vi "运维调试_氨氮.vi"() -> ()   [LabVIEW 2016, in "氨氮.lvlib"]
uses:
  <vilib>/Platform/TimedLoop/XDataNode/timing_clust.ctl
  <vilib>/Platform/TimedLoop/XDataNode/nitl_modes.ctl
  <vilib>/Platform/TimedLoop/XDataNode/wakeup.ctl
  <vilib>/Utility/miscctls.llb/LVPointTypeDef.ctl
  <vilib>/Platform/TimedLoop/XDataNode/XDataNode.xnode
  <vilib>/Platform/TimedLoop/XDataNode/XDNodeRunTimeDep.lvlib
panel:
  out "固件版本号":string
  in  "数组":string[](array[string])
  in  "备用系数写入":bool
  in  "备用系数读取":bool
  in  "备用系数":T1
  in  "量程切换阈值写入":bool
  in  "量程切换阈值读取":bool
  in  "量程切换阈值":cluster{"阈值":dbl, "标液浓度":dbl}
  in  "参数下拉列表":enum16{"氨氮", "总磷"}(ring)
  in  "量程下拉列表":enum16{"低量程", "高量程"}(ring)
  in  "测量模式下拉列表":enum16{"水样测量", "空白核查", "标样核查", "盲样测试", "加标回收"}(ring)
  in  "公式":cluster{"X^2":dbl, "X":dbl, "b":dbl}
  in  "写公式":bool
  in  "读公式":bool
  in  "精度":dbl=4.0
  in  "样品5 F0":dbl
  in  "样品5 F1":dbl
  in  "样品4 F1":dbl
  in  "样品4 F0":dbl
  in  "样品3 F0":dbl
  in  "样品3 F1":dbl
  in  "样品2 F0":dbl
  in  "样品2 F1":dbl
  in  "样品1 F1":dbl
  in  "样品1 F0":dbl
  in  "method":u16(ring) items=["最小二乘", "最小绝对残差", "Bisquare"]
  in  "模型":enum32{"线性", "多项式"}(ring)
  out "r^2":dbl format="%.7g"
  out "拟合公式":string
  in  "样品2启用":bool
  in  "样品5启用":bool
  in  "样品4启用":bool
  in  "样品3启用":bool
  in  "样品1启用":bool
  in  "标液浓度5":dbl
  in  "测量吸光度5":dbl
  in  "标液浓度4":dbl
  in  "测量吸光度4":dbl
  in  "标液浓度3":dbl
  in  "测量吸光度3":dbl
  in  "标液浓度2":dbl
  in  "测量吸光度2":dbl
  in  "测量吸光度1":dbl
  in  "标液浓度1":dbl
  out "XY图":cluster{"X Values":dbl[], "Y Values":dbl[]}[](graph)
  in  "返回":bool
  in  "设置":bool
  out "序列号":string="序列号"
  out "氨氮测量数据":T2(xcontrol)
  out "集成报警信息":string
  out "设置值":dbl
  out "定时启动":bool
  out "总磷总氮运行状态":T3(xcontrol)
  in  "停止":bool
  in  "手动启动":bool
  in  "单步测试":bool
  in  "总磷氨氮调试":u16[](xcontrol)
  out "F3":sgl format="%#.6f"
  out "F2":sgl format="%#.6f"
  out "F1":sgl format="%#.6f"
  out "F0":sgl format="%#.6f"
  out "多列列表框":i32(listbox)
  # "COM6"
  # "参数设置"
  # "标液浓度"
  # "F0"
  # "F1"
  # "吸光值显示"
  # "样品一"
  # "辅\n助\n计\n算\n区"
  # "样品二"
  # "样品三"
  # "样品四"
  # "样品五"
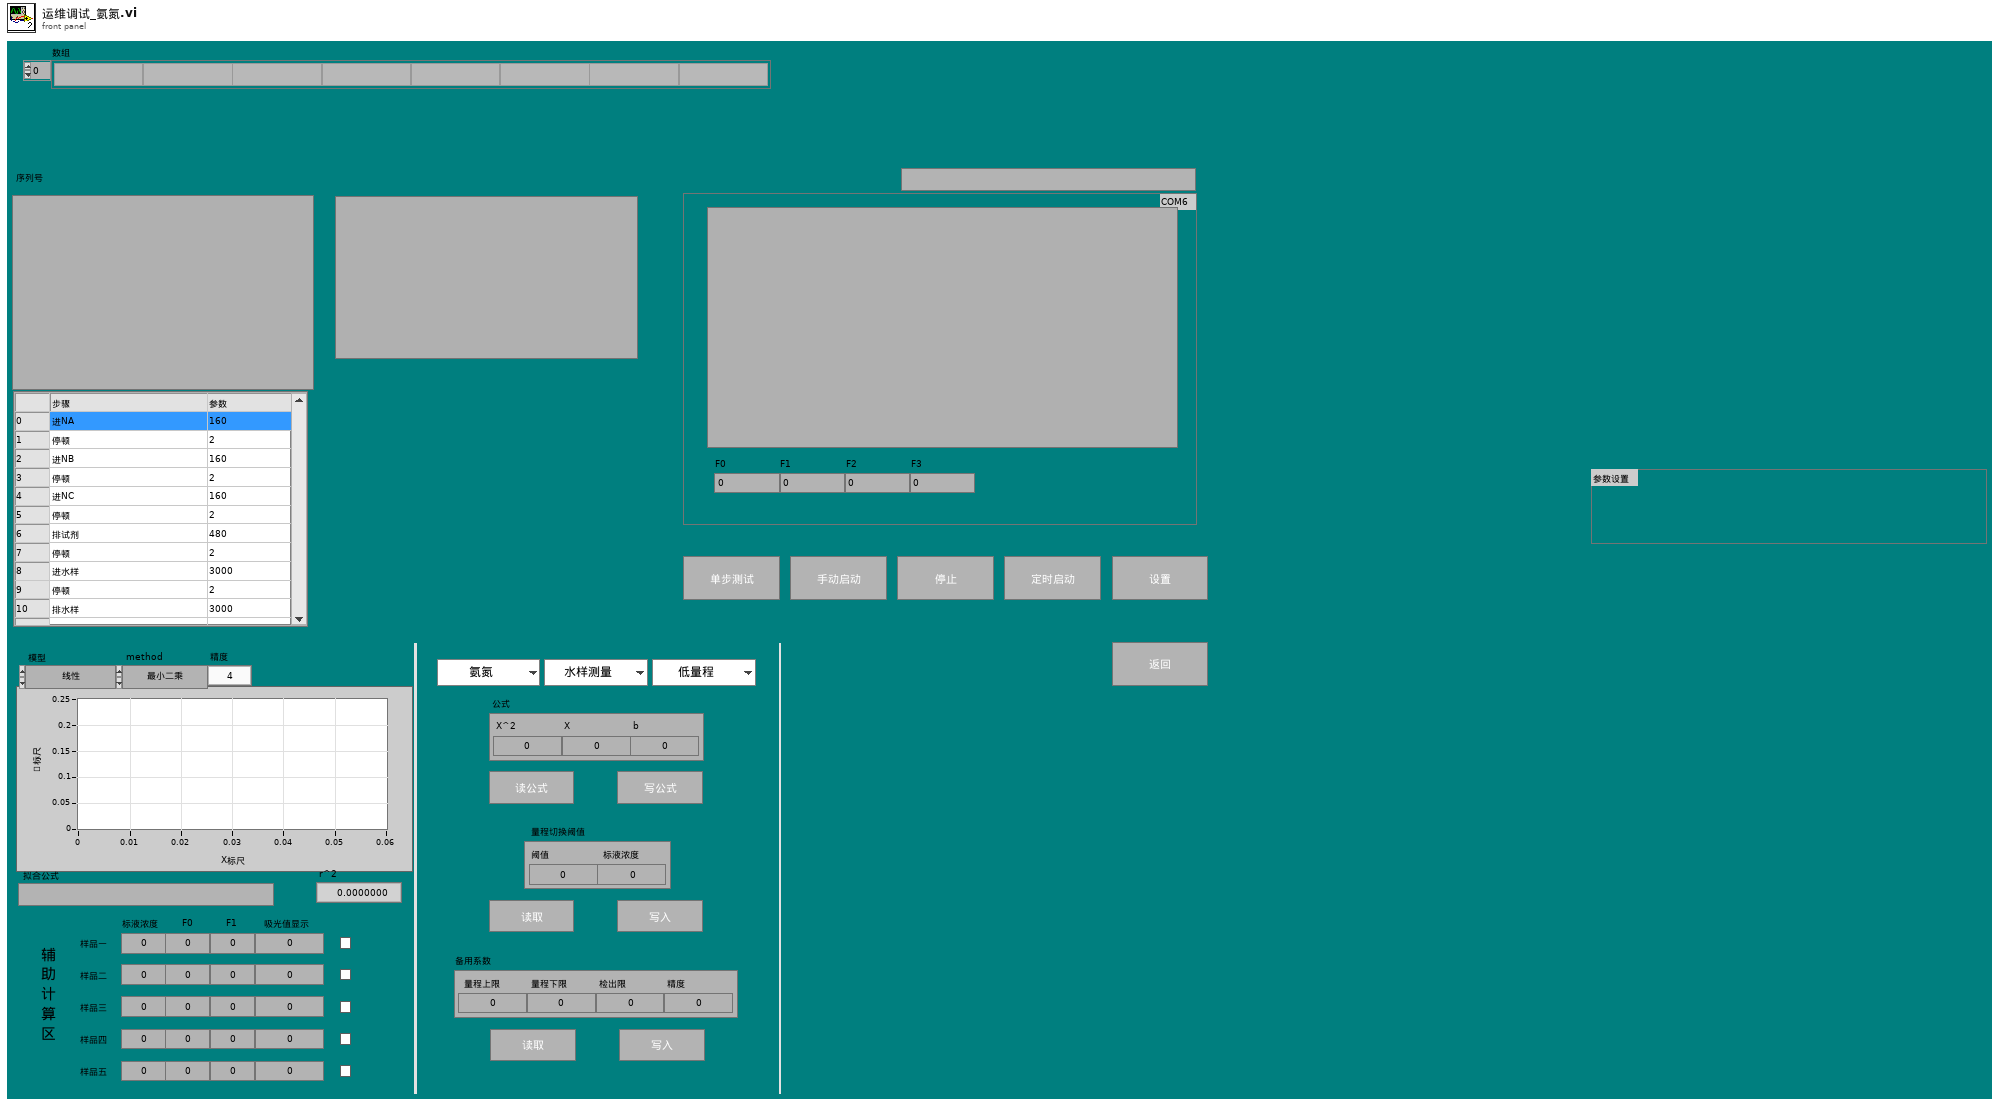
[diagram p1: front panel]
types:
  T1 = cluster{"量程上限":dbl, "量程下限":dbl, "检出限":dbl, "精度":dbl}
  T2 = cluster{"flowid":u16, "测量精度":u16, "测量数据区":cluster{"因子编码":u32, "单位":u16, "标样参考值":sgl, "水样数据时间":timestamp, "水样实测值":sgl, "水样数据标识":string, "标样数据时间":timestamp, "标样实测值":sgl, "标样数据标识":string, "空白数据时间":timestamp, "空白实测值":sgl, "空白数据标识":string, "零点核查数据时间":timestamp, "零点核查实测值":sgl, "零点核查数据标识":string, "跨度核查数据时间":timestamp, "跨度核查实测值":sgl, "跨度核查数据标识":string, "加标回收数据时间":timestamp, "加标回收实测值":sgl, "加标回收数据标识":string, "平行样数据时间":timestamp, "平行样实测值":sgl, "平行样数据标识":string}}
  T3 = cluster{"系统时间":timestamp, "工作状态":enum16{"空闲", "水样测试", "标样核查", "零点核查", "跨度核查", "空白测试", "平行样测试", "加标回收", "空白校准", "标样校准", "初始化（清洗）"}, "测量模式":enum16{"待机", "连续模式", "周期模式", "定点模式", "受控模式", "手动模式"}, "告警代码":enum16{"无告警", "缺试剂告警", "缺水样告警", "缺蒸馏水告警", "缺标液告警", "仪表漏液告警", "标定异常告警", "超量程告警", "加热异常", "低试剂预警", "超上限告警", "超下限告警", "仪表内部其他异常", "滴定异常告警", "电极异常告警", "量程切换告警", "参数设置告警", "PH电极电位异常", "电导率电极异常", "浊度光度异常", "溶解氧电极异常", "溶解氧光强异常", "温度异常告警", "PH异常告警", "溶解氧异常告警", "电导率异常告警", "浊度异常告警", "叶绿素异常告警", "藻密度异常告警", "蓝绿藻异常告警", "ORP异常告警", "氨氮异常告警", "清洁刷异常告警", "SD卡异常告警", "蓝牙异常告警", "Wifi异常告警", "流程异常告警"}, "故障代码":enum16{"无故障", "电机故障", "温度故障", "通讯故障", "滴定故障"}, "日志代码":u16, "软件版本":u16, "F0":sgl, "F1":sgl, "F2":sgl, "F3":sgl, "T":sgl, "H":sgl, "id":u16, "flowid":u16, "量程":u16}
  T4 = enum16{"待机", "启动氨氮", "氨氮测量中", "启动总磷", "总磷测量中", "延时"}
  T5 = typedef "LVPointTypeDef.ctl" = cluster{"Horizontal":i16, "Vertical":i16}
  T6 = cluster{"因子编码":u32, "单位":u16, "标样参考值":sgl, "水样数据时间":timestamp, "水样实测值":sgl, "水样数据标识":string, "标样数据时间":timestamp, "标样实测值":sgl, "标样数据标识":string, "空白数据时间":timestamp, "空白实测值":sgl, "空白数据标识":string, "零点核查数据时间":timestamp, "零点核查实测值":sgl, "零点核查数据标识":string, "跨度核查数据时间":timestamp, "跨度核查实测值":sgl, "跨度核查数据标识":string, "加标回收数据时间":timestamp, "加标回收实测值":sgl, "加标回收数据标识":string, "平行样数据时间":timestamp, "平行样实测值":sgl, "平行样数据标识":string}
  T7 = enum16{"空闲", "水样测试", "标样核查", "零点核查", "跨度核查", "空白测试", "平行样测试", "加标回收", "空白校准", "标样校准", "初始化（清洗）"}
  T8 = cluster{"启动模式":enum16{"标液测量", "水样测量", "零液测量", "盲样测量", "加标回收"}, "启动参数":u16, "量程":enum16{"低量程", "高量程"}}
  T9 = cluster{"时间标识":timestamp, "设备":string, "日志信息":string, "流程参数":string}
  T10 = cluster{"时间标识":timestamp, "设备":string, "日志信息":string}
  T11 = enum16{"无告警", "缺试剂告警", "缺水样告警", "缺蒸馏水告警", "缺标液告警", "仪表漏液告警", "标定异常告警", "超量程告警", "加热异常", "低试剂预警", "超上限告警", "超下限告警", "仪表内部其他异常", "滴定异常告警", "电极异常告警", "量程切换告警", "参数设置告警", "PH电极电位异常", "电导率电极异常", "浊度光度异常", "溶解氧电极异常", "溶解氧光强异常", "温度异常告警", "PH异常告警", "溶解氧异常告警", "电导率异常告警", "浊度异常告警", "叶绿素异常告警", "藻密度异常告警", "蓝绿藻异常告警", "ORP异常告警", "氨氮异常告警", "清洁刷异常告警", "SD卡异常告警", "蓝牙异常告警", "Wifi异常告警", "流程异常告警"}
  T12 = typedef "LVRowAndColumnUnsignedTypeDef.ctl" = cluster{"Row":u32, "Column":u32}
  T13 = typedef "XDNodeRunTimeDep.lvlib/timing_clust.ctl" = cluster{"Expected End [f-1]":u64, "Actual End [f-1]":u64, "Finished Late? [f-1]":bool, "Expected End [i-1]":u64, "Actual End [i-1]":u64, "Finished Late? [i-1]":bool, "Expected Start [i]":u64, "Actual Start [i]":u64, "Expected Start [f]":u64, "Actual Start [f]":u64, "Source Name":string, "Structure Name":string, "Period":i64, "Deadline":i64, "Offset":i64, "Start":i64, "Priority":i32, "Timeout":i32, "Mode":T14, "Wakeup Reason":T15, "Error":errorcluster, "Source Type":string, "Secondary Source Type":string, "Global End Time":u64, "Global Start Time":u64, "Frame Duration":u64, "Iteration Duration":u64, "Assigned CPU":i32, "I/O Scan Engine Mode":u32}
  T14 = typedef "XDNodeRunTimeDep.lvlib/nitl_modes.ctl" = enum32{"No Change", "Process missed periods, maintain original phase", "Discard missed periods, maintain original phase", "Process missed periods, ignore original phase", "Discard missed periods, ignore original phase"}
  T15 = typedef "XDNodeRunTimeDep.lvlib/wakeup.ctl" = enum32{"Normal", "Aborted", "Asynchronous wakeup", "Timing source error", "Timed loop error", "Timeout"}
  T16 = cluster{"站号":u16, "量程切换":enum32{"H", "L", "AUTO"}, "控制命令":enum16{"启动测量", "标样核查", "零点核查", "跨度核查", "空白测试", "平行样测试", "加标回收", "空白校准", "标样校准", "初始化（清洗）", "停止测试", "仪器重启", "校时", "模式设置", "测量间隔设置", "盲样测试"}, "模式设置":enum16{"待机", "连续模式", "周期模式", "定点模式", "受控模式", "手动模式"}, "测量间隔":u16}
  T17 = cluster{"站号":u16, "量程切换":enum32{"H", "L", "AUTO"}, "控制命令":enum16{"启动测量", "标样核查", "零点核查", "跨度核查", "空白测试", "平行样测试", "加标回收", "空白校准", "标样校准", "初始化（清洗）", "停止测试", "仪器重启", "校时", "模式设置", "测量间隔设置"}, "模式设置":enum16{"待机", "连续模式", "周期模式", "定点模式", "受控模式", "手动模式"}, "测量间隔":u16}
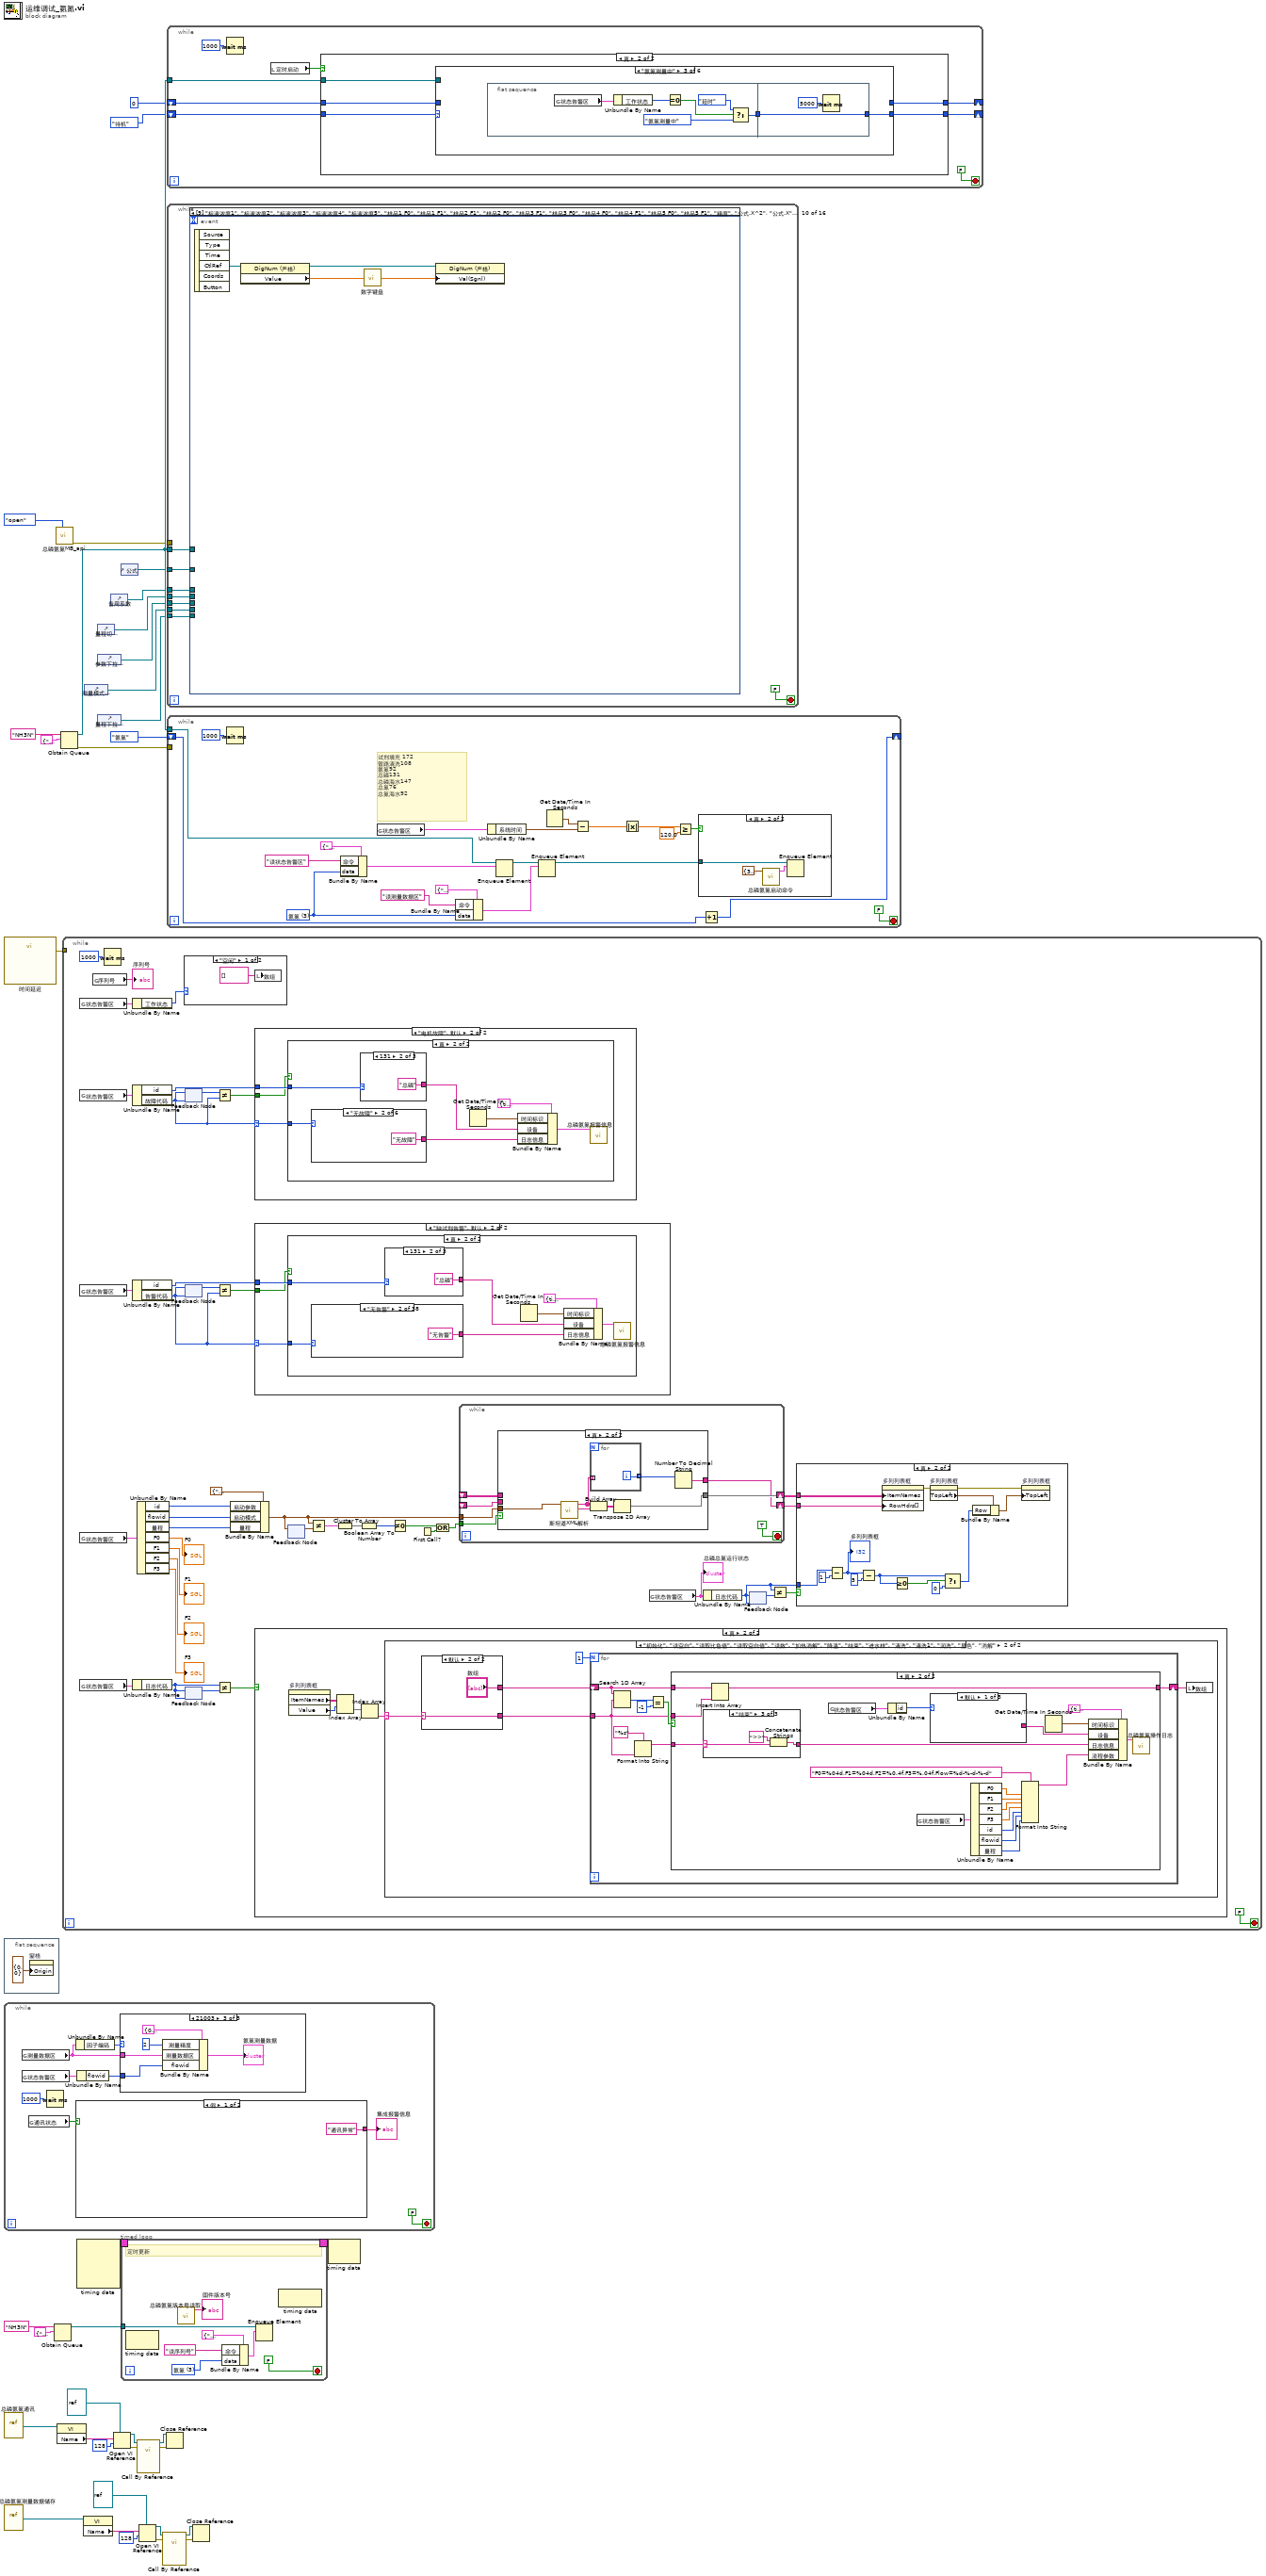
[diagram p0: block diagram]
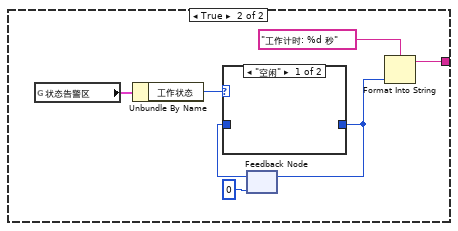
[diagram p2: hidden frame]
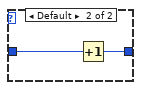
[diagram p3: hidden frame]
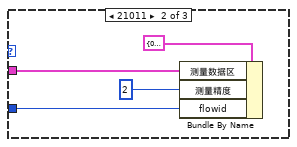
[diagram p5: hidden frame]
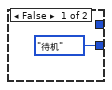
[diagram p6: hidden frame]
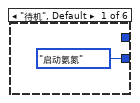
[diagram p7: hidden frame]
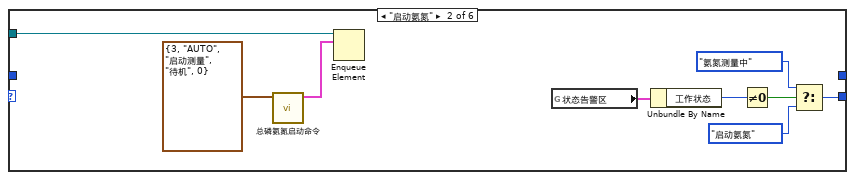
[diagram p8: hidden frame]
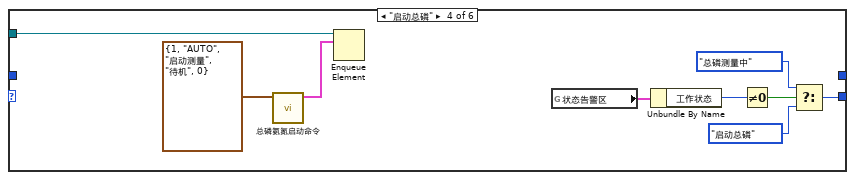
[diagram p9: hidden frame]
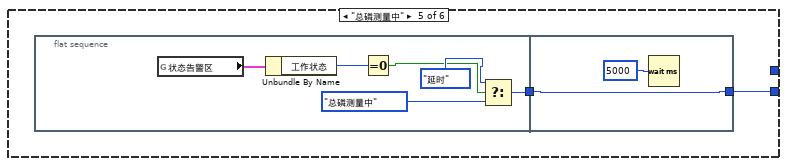
[diagram p10: hidden frame]
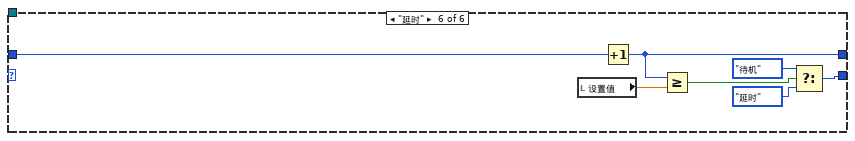
[diagram p11: hidden frame]
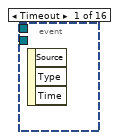
[diagram p12: hidden frame]
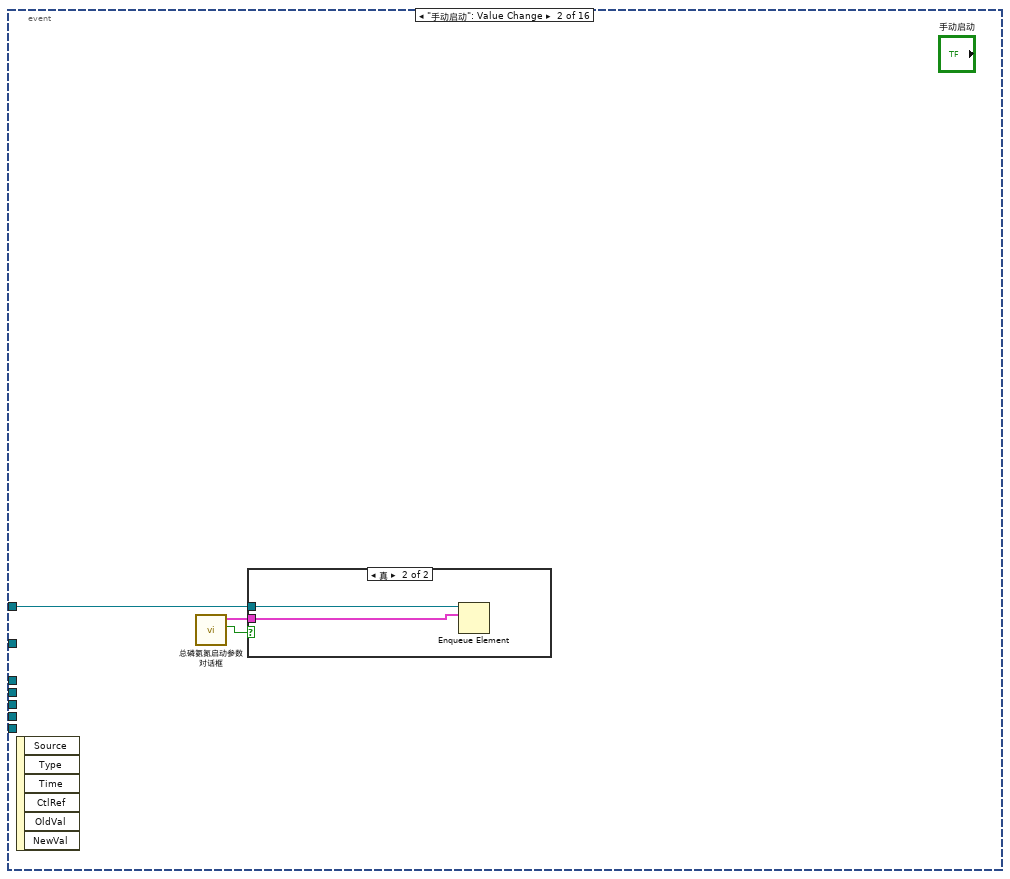
[diagram p13: hidden frame]
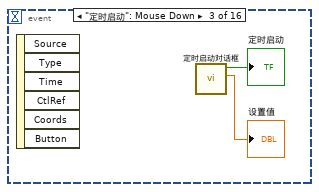
[diagram p15: hidden frame]
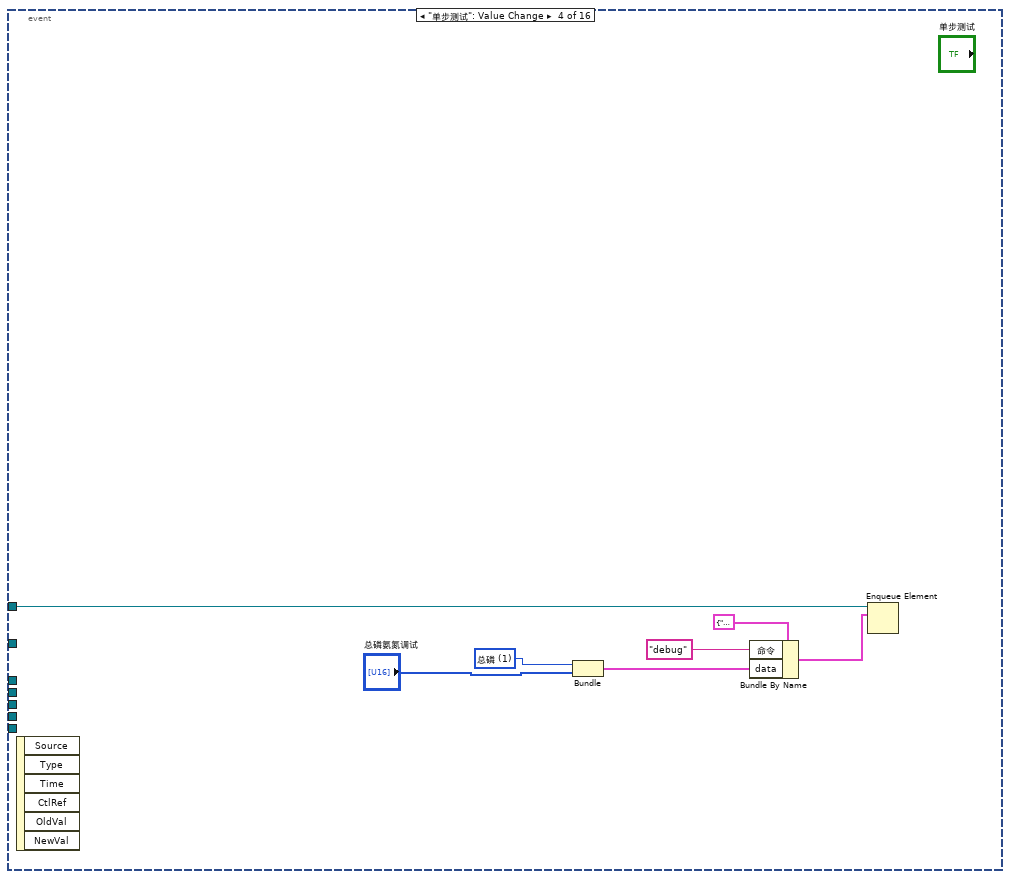
[diagram p16: hidden frame]
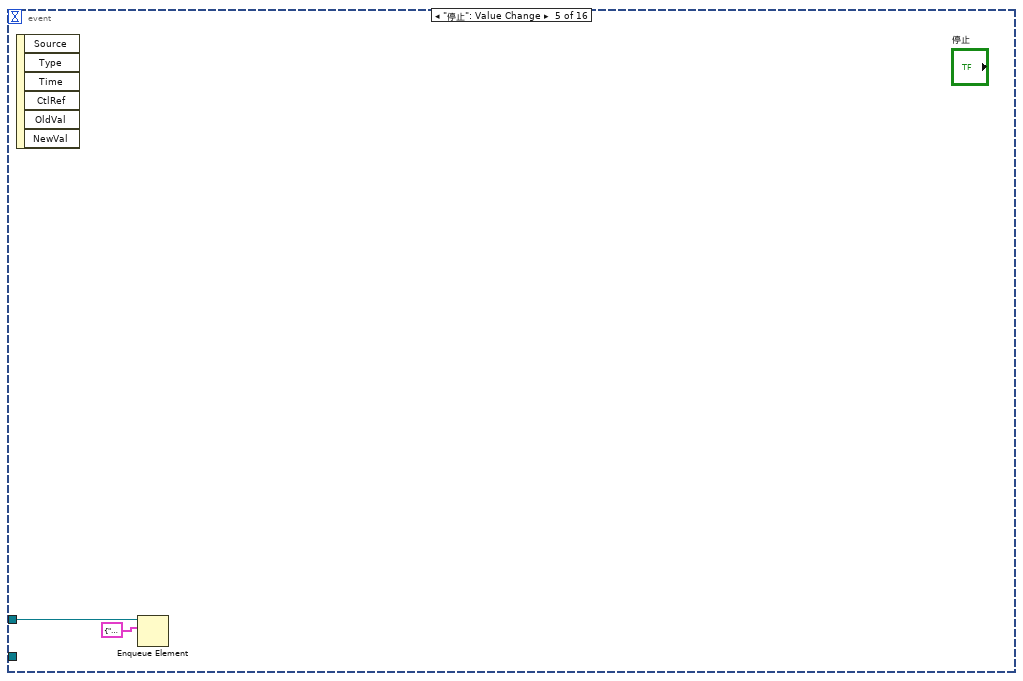
[diagram p17: hidden frame]
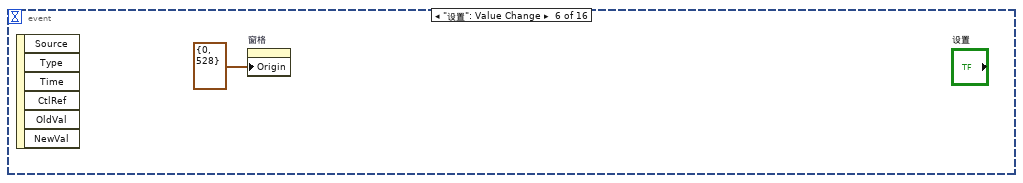
[diagram p18: hidden frame]
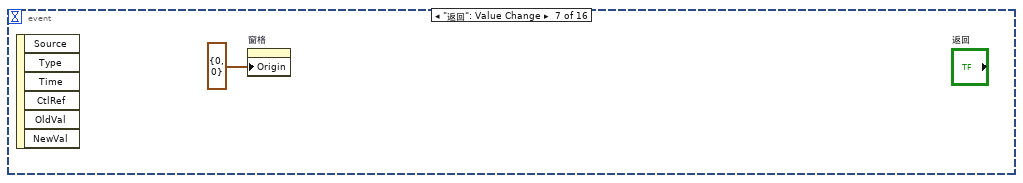
[diagram p19: hidden frame]
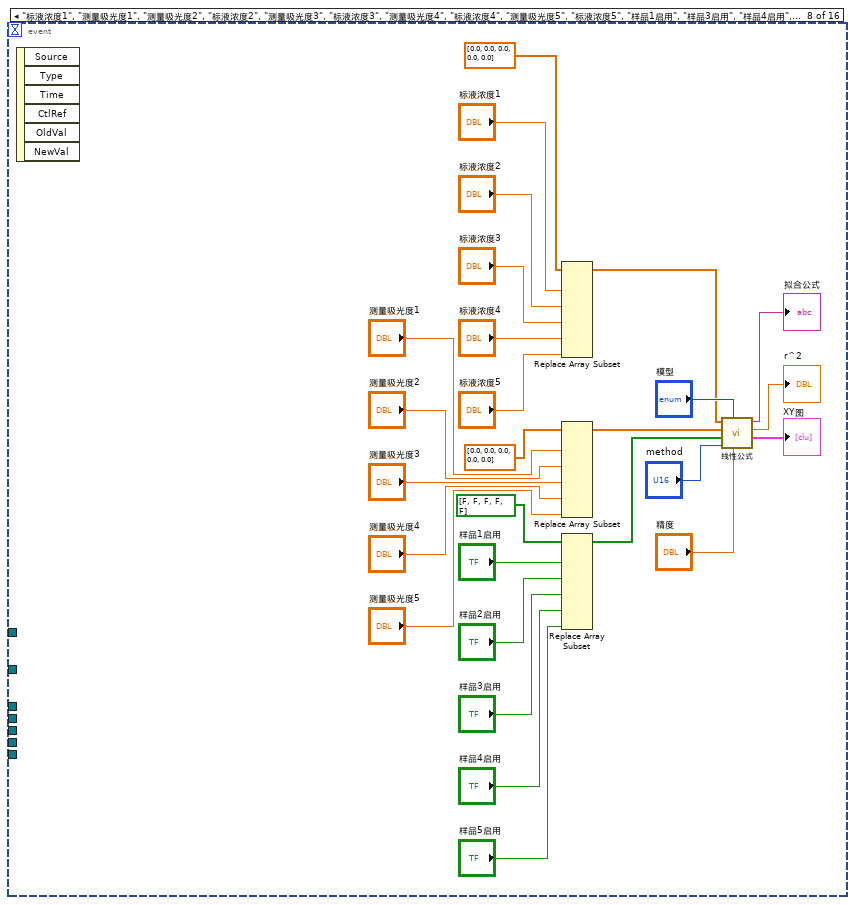
[diagram p20: hidden frame]
diagram:
  n1 = call "时间延迟"() -> ("error out"=w8:errorcluster)  [unwired: 11 in]
  n2 = flat-sequence {
    frame #0 {
      n3 = property on="窗格" class="Pane"("Origin"=T5 {"Horizontal"=0, "Vertical"=0} ("原点")) -> ()  [unwired: 2 in, 2 out]
    }
  }
  n4 = while {
    stop <- FALSE stop-if-true
    n5 = global read "VAR总磷氨氮全局变量.vi" "测量数据区"() -> (w44:T6)
    n6 = global read "VAR总磷氨氮全局变量.vi" "状态告警区"() -> (w40:T3)
    n7 = global read "VAR总磷氨氮全局变量.vi" "通讯状态"() -> (w42:bool)
    n8 = Wait (ms)(milliseconds to wait=u32 1000 ("等待时间（毫秒）")) -> ()  [unwired: 1 out]
    n9 = Unbundle By Name(w44) -> ("因子编码"=w43:u32)
    n10 = case shown="假" w42 {
      tunnel: ["通讯异常" ("集成报警信息") w48] -> w41
      frame False {
      }
      frame True {
        n11 = global read "VAR总磷氨氮全局变量.vi" "状态告警区"() -> (w54:T3)
        n12 = Unbundle By Name(w54) -> ("工作状态"=w53:T7)
        n13 = feedback #1(0) -> (w51:i32)
        n14 = case shown="\"空闲\"" w53 {
          tunnel: w51 -> [_ w56]
          tunnel: [_ w55] -> w49
          frame "空闲" {
          }
          frame Default {
            n15 = Increment(x=w56) -> (x+1=w55:i32)
          }
        }
        n16 = feedback-in #1(w49) -> ()
        n17 = Format Into String(format string="工作计时: %d 秒" ("格式字符串"), w49) -> (resulting string=w48:string)  [unwired: 2 in, 1 out]
      }
    }
    "集成报警信息" <- w41
    n18 = Unbundle By Name(w40) -> ("flowid"=w39:u16)
    n19 = case shown="21003" w43 {
      tunnel: w44 -> [_ w60 w65]
      tunnel: w39 -> [_ w58 w63]
      frame Default {
      }
      frame 21011 {
        n20 = Bundle By Name(cluster=T2 {"flowid"=0, "测量精度"=0, "测量数据区"={"因子编码"=0, "单位"=0, "标样参考值"=0.0, "水样数据时间"=timestamp(0 s since 1904-01-01), "水样实测值"=0.0, "水样数据标识"="", "标样数据时间"=timestamp(0 s since 1904-01-01), "标样实测值"=0.0, "标样数据标识"="", "空白数据时间"=timestamp(0 s since 1904-01-01), "空白实测值"=0.0, "空白数据标识"="", "零点核查数据时间"=timestamp(0 s since 1904-01-01), "零点核查实测值"=0.0, "零点核查数据标识"="", "跨度核查数据时间"=timestamp(0 s since 1904-01-01), "跨度核查实测值"=0.0, "跨度核查数据标识"="", "加标回收数据时间"=timestamp(0 s since 1904-01-01), "加标回收实测值"=0.0, "加标回收数据标识"="", "平行样数据时间"=timestamp(0 s since 1904-01-01), "平行样实测值"=0.0, "平行样数据标识"=""}} ("氨氮测量数据"), "测量数据区"=w60, "测量精度"=u16 2, "flowid"=w58) -> ()  [unwired: 1 out]
      }
      frame 21003 {
        n21 = Bundle By Name(cluster=T2 {"flowid"=0, "测量精度"=0, "测量数据区"={"因子编码"=0, "单位"=0, "标样参考值"=0.0, "水样数据时间"=timestamp(0 s since 1904-01-01), "水样实测值"=0.0, "水样数据标识"="", "标样数据时间"=timestamp(0 s since 1904-01-01), "标样实测值"=0.0, "标样数据标识"="", "空白数据时间"=timestamp(0 s since 1904-01-01), "空白实测值"=0.0, "空白数据标识"="", "零点核查数据时间"=timestamp(0 s since 1904-01-01), "零点核查实测值"=0.0, "零点核查数据标识"="", "跨度核查数据时间"=timestamp(0 s since 1904-01-01), "跨度核查实测值"=0.0, "跨度核查数据标识"="", "加标回收数据时间"=timestamp(0 s since 1904-01-01), "加标回收实测值"=0.0, "加标回收数据标识"="", "平行样数据时间"=timestamp(0 s since 1904-01-01), "平行样实测值"=0.0, "平行样数据标识"=""}} ("氨氮测量数据"), "测量精度"=u16 2, "测量数据区"=w65, "flowid"=w63) -> (→"氨氮测量数据":T2)
      }
    }
  }
  n22 = vi-ref "总磷氨氮通讯.vi"() -> (w31:refnum<vi>)
  n23 = vi-ref "总磷氨氮测量数据储存.vi"() -> (w23:refnum<vi>)
  n24 = Obtain Queue(name (unnamed)="NH3N" ("名称（未命名）"), element data type=cluster{"命令":string, "data":variant} {"命令"="", "data"=variant}) -> (queue out=w1:refnum<queue>)  [unwired: 3 in, 2 out]
  n25 = call "总磷氨氮MB_api.vi"("STEP"=enum16{"open", "read", "write", "close"}."open") -> ("error out"=w7:errorcluster)  [unwired: 8 in, 2 out]
  n26 = property class="VI"(reference=w31) -> ("Name"=w30:string)  [unwired: 1 in, 2 out]
  n27 = Obtain Queue(name (unnamed)="NH3N" ("名称（未命名）"), element data type=cluster{"命令":string, "data":variant} {"命令"="", "data"=variant}) -> (queue out=w34:refnum<queue>, error out=w35:errorcluster)  [unwired: 3 in, 1 out]
  n28 = while {
    tunnel: w8 -> [_]
    stop <- FALSE stop-if-true
    n29 = global read "VAR总磷氨氮全局变量.vi" "状态告警区"() -> (w71:T3)
    n30 = global read "VAR总磷氨氮全局变量.vi" "状态告警区"() -> (w77:T3)
    n31 = global read "VAR总磷氨氮全局变量.vi" "状态告警区"() -> (w82:T3)
    n32 = global read "VAR总磷氨氮全局变量.vi" "状态告警区"() -> (w94:T3)
    n33 = global read "VAR总磷氨氮全局变量.vi" "状态告警区"() -> (w68:T3)
    n34 = global read "VAR总磷氨氮全局变量.vi" "序列号"() -> (→"序列号":string)
    n35 = Wait (ms)(milliseconds to wait=u32 1000 ("等待时间（毫秒）")) -> ()  [unwired: 1 out]
    n36 = Unbundle By Name(w71) -> ("工作状态"=w70:T7)
    n37 = Unbundle By Name(w77) -> ("id"=w76:u16, "故障代码"=w73:enum16{"无故障", "电机故障", "温度故障", "通讯故障", "滴定故障"})
    n38 = Unbundle By Name(w82) -> ("id"=w81:u16, "告警代码"=w78:T11)
    n39 = Unbundle By Name(w68) -> ("日志代码"=w67:u16)
    n40 = Unbundle By Name(w94) -> ("id"=w91:u16, "flowid"=w93:u16, "量程"=w92:u16, "F0"=→"F0":sgl, "F1"=→"F1":sgl, "F2"=→"F2":sgl, "F3"=→"F3":sgl)
    n41 = case shown="\"空闲\"" w70 {
      frame "空闲" {
        n42 = local write "数组"(string[] [] ("数组")) -> ()
      }
      frame "水样测试", Default {
      }
    }
    n43 = feedback #2(w73) -> (w74:enum16{"无故障", "电机故障", "温度故障", "通讯故障", "滴定故障"})
    n44 = feedback-in #2(w73) -> ()
    n45 = feedback #3(w78) -> (w79:T11)
    n46 = feedback-in #3(w78) -> ()
    n47 = feedback #4(w67) -> (w69:u16)
    n48 = feedback-in #4(w67) -> ()
    n49 = Not Equal?(x=w74, y=w73) -> (x != y?=w75:bool)
    n50 = Not Equal?(x=w79, y=w78) -> (x != y?=w80:bool)
    n51 = Not Equal?(x=w67, y=w69) -> (x != y?=w66:bool)
    n52 = Bundle By Name(cluster=T8 {"启动模式"=enum."加标回收", "启动参数"=1, "量程"=enum."低量程"} ("参数簇"), "启动参数"=w91, "启动模式"=w93, "量程"=w92) -> (w84:T8)
    n53 = case shown="\"电机故障\", 默认" w73 {
      selector: w73 -> [_ w162]
      tunnel: w76 -> [_ w163]
      tunnel: w75 -> [_ w161]
      frame "无故障" {
      }
      frame "电机故障", Default {
        n54 = case shown="真" w161 {
          tunnel: w163 -> [_ w170]
          tunnel: w162 -> [_ w165]
          frame False {
          }
          frame True {
            n55 = case shown="\"无故障\"" w165 {
              selector: w165 -> [w172 _ _ _ _ _]
              tunnel: [w171 "无故障" "电机故障" "温度故障" "通讯故障" "滴定故障"] -> w164
              frame Default {
                n56 = Format Into String(format string="%d" ("格式字符串"), initial string="未知" ("工作状态"), w172) -> (resulting string=w171:string)  [unwired: 1 in, 1 out]
              }
              frame "无故障" {
              }
              frame "电机故障" {
              }
              frame "温度故障" {
              }
              frame "通讯故障" {
              }
              frame "滴定故障" {
              }
            }
            n57 = case shown="131" w170 {
              tunnel: [_ "总磷" ("table输入") "氨氮" ("table输入")] -> w166
              frame Default {
              }
              frame 131 {
              }
              frame 92 {
              }
            }
            n58 = Get Date/Time In Seconds() -> (seconds since 1Jan1904=w167:timestamp)
            n59 = Bundle By Name(cluster=T10 {"时间标识"=timestamp(0 s since 1904-01-01), "设备"="", "日志信息"=""} ("data in"), "时间标识"=w167, "设备"=w166, "日志信息"=w164) -> (w168:T10)
            n60 = call "总磷氨氮报警信息.vi"("data in"=w168) -> ()  [unwired: 11 in]
          }
        }
      }
    }
    n61 = case shown="\"缺试剂告警\", 默认" w78 {
      selector: w78 -> [_ w183]
      tunnel: w81 -> [_ w184]
      tunnel: w80 -> [_ w182]
      frame "无告警" {
      }
      frame "缺试剂告警", Default {
        n62 = case shown="真" w182 {
          tunnel: w184 -> [_ w191]
          tunnel: w183 -> [_ w185]
          frame False {
          }
          frame True {
            n63 = case shown="\"无告警\"" w185 {
              selector: w185 -> [w193 _ _ _ _ _ _ _ _ _ _ _ _ _ _ _ _ _ _ _ _ _ _ _ _ _ _ _ _ _ _ _ _ _ _ _ _ _]
              tunnel: [w192 "无告警" "缺试剂告警" "缺水样告警" "缺蒸馏水告警" "缺标液告警" "仪表漏液告警" "标定异常告警" "超量程告警" "加热异常" "低试剂预警" "超上限告警" "超下限告警" "仪表内部其他异常" "滴定异常告警" "电极异常告警" "量程切换告警" "参数设置告警" "PH电极电位异常" "电导率电极异常" "浊度光度异常" "溶解氧电极异常" "溶解氧光强异常" "温度异常告警" "PH异常告警" "溶解氧异常告警" "电导率异常告警" "浊度异常告警" "叶绿素异常告警" "藻密度异常告警" "蓝绿藻异常告警" "ORP异常告警" "氨氮异常告警" "清洁刷异常告警" "SD卡异常告警" "蓝牙异常告警" "WiFi异常告警" "流程异常告警"] -> w186
              frame Default {
                n64 = Format Into String(format string="%d" ("格式字符串"), initial string="未知" ("工作状态"), w193) -> (resulting string=w192:string)  [unwired: 1 in, 1 out]
              }
              frame "无告警" {
              }
              frame "缺试剂告警" {
              }
              frame "缺水样告警" {
              }
              frame "缺蒸馏水告警" {
              }
              frame "缺标液告警" {
              }
              frame "仪表漏液告警" {
              }
              frame "标定异常告警" {
              }
              frame "超量程告警" {
              }
              frame "加热异常" {
              }
              frame "低试剂预警" {
              }
              frame "超上限告警" {
              }
              frame "超下限告警" {
              }
              frame "仪表内部其他异常" {
              }
              frame "滴定异常告警" {
              }
              frame "电极异常告警" {
              }
              frame "量程切换告警" {
              }
              frame "参数设置告警" {
              }
              frame "PH电极电位异常" {
              }
              frame "电导率电极异常" {
              }
              frame "浊度光度异常" {
              }
              frame "溶解氧电极异常" {
              }
              frame "溶解氧光强异常" {
              }
              frame "温度异常告警" {
              }
              frame "PH异常告警" {
              }
              frame "溶解氧异常告警" {
              }
              frame "电导率异常告警" {
              }
              frame "浊度异常告警" {
              }
              frame "叶绿素异常告警" {
              }
              frame "藻密度异常告警" {
              }
              frame "蓝绿藻异常告警" {
              }
              frame "ORP异常告警" {
              }
              frame "氨氮异常告警" {
              }
              frame "清洁刷异常告警" {
              }
              frame "SD卡异常告警" {
              }
              frame "蓝牙异常告警" {
              }
              frame "Wifi异常告警" {
              }
              frame "流程异常告警" {
              }
            }
            n65 = case shown="131" w191 {
              tunnel: [_ "总磷" ("table输入") "氨氮" ("table输入")] -> w187
              frame Default {
              }
              frame 131 {
              }
              frame 92 {
              }
            }
            n66 = Get Date/Time In Seconds() -> (seconds since 1Jan1904=w188:timestamp)
            n67 = Bundle By Name(cluster=T10 {"时间标识"=timestamp(0 s since 1904-01-01), "设备"="", "日志信息"=""} ("data in"), "时间标识"=w188, "设备"=w187, "日志信息"=w186) -> (w189:T10)
            n68 = call "总磷氨氮报警信息.vi"("data in"=w189) -> ()  [unwired: 11 in]
          }
        }
      }
    }
    n69 = case shown="真" w66 {
      frame False {
      }
      frame True {
        n70 = property on="多列列表框" class="MCListbox (严格)"() -> ("ItemNames"=w111:string[][], "Value"=w112:i32)  [unwired: 2 in, 2 out]
        n71 = Index Array(array=w111, index (row)=w112) -> (element=w110:string[])  [unwired: 1 in]
        n72 = Index Array(array=w110) -> (element=w109:string)  [unwired: 1 in]
        n73 = case shown="\"初始化\", \"读空白\", \"读取比色值\", \"读取空白值\", \"读数\", \"加热消解\", \"降温\", \"结束\", \"进水样\", \"清洗\", \"清洗1\", \"润洗\", \"显色\", \"消解\"" w109 {
          selector: w109 -> [_ w115]
          frame Default {
          }
          frame "初始化", "读空白", "读取比色值", "读取空白值", "读数", "加热消解", "降温", "结束", "进水样", "清洗", "清洗1", "润洗", "显色", "消解" {
            n74 = case shown="默认" w115 {
              selector: w115 -> [w119 w121]
              tunnel: [w119 w121] -> w114
              tunnel: [string[] [] ("数组") "数组"] -> w113
              frame "读数" {
              }
              frame Default {
              }
            }
            n75 = for {
              N: 1 -> [_]
              tunnel: w114 -> [w123]
              shift-right: [w122] -> w116
              shift-left: w113 -> [w124]
              n76 = Search 1D Array(1D array=w124, element=w123) -> (index of element=w127:i32)  [unwired: 1 in]
              n77 = Format Into String(format string="%s" ("格式字符串"), w123) -> (resulting string=w128:string)  [unwired: 2 in, 1 out]
              n78 = Equal?(x=w127, y=-1) -> (x = y?=w125:bool)
              n79 = case shown="真" w125 {
                tunnel: w128 -> [_ w132]
                tunnel: w124 -> [w130 w136]
                tunnel: w123 -> [_ w135]
                tunnel: [w130 w134] -> w122
                frame False {
                }
                frame True {
                  n80 = case shown="\"结束\"" w132 {
                    selector: w132 -> [w152 w155 w158]
                    tunnel: [w152 w154 w157] -> w131
                    frame Default {
                    }
                    frame "初始化" {
                      n81 = Concatenate Strings("<<" ("字符串"), w155) -> (w154:string)
                    }
                    frame "结束" {
                      n82 = Concatenate Strings(">>" ("字符串"), w158) -> (w157:string)
                    }
                  }
                  n83 = Insert Into Array(array=w136, new element=w135) -> (w134:string[])  [unwired: 1 in]
                  n84 = global read "VAR总磷氨氮全局变量.vi" "状态告警区"() -> (w151:T3)
                  n85 = Unbundle By Name(w151) -> ("id"=w150:u16)
                  n86 = global read "VAR总磷氨氮全局变量.vi" "状态告警区"() -> (w146:T3)
                  n87 = case shown="默认" w150 {
                    tunnel: [_ "总磷" ("table输入") "氨氮" ("table输入")] -> w148
                    frame Default {
                    }
                    frame 131 {
                    }
                    frame 92 {
                    }
                  }
                  n88 = Unbundle By Name(w146) -> ("F0"=w143:sgl, "F1"=w142:sgl, "F2"=w141:sgl, "F3"=w140:sgl, "id"=w139:u16, "flowid"=w138:u16, "量程"=w137:u16)
                  n89 = Format Into String(format string="F0=%04d,F1=%04d,F2=%0.4f,F3=%.04f,Flow=%d-%-d-%-d" ("格式字符串"), w143, w142, w141, w140, w139, w138, w137) -> (resulting string=w144:string)  [unwired: 2 in, 1 out]
                  n90 = Get Date/Time In Seconds() -> (seconds since 1Jan1904=w147:timestamp)
                  n91 = Bundle By Name(cluster=T9 {"时间标识"=timestamp(0 s since 1904-01-01), "设备"="", "日志信息"="", "流程参数"=""} ("data in"), "时间标识"=w147, "设备"=w148, "日志信息"=w131, "流程参数"=w144) -> (w149:T9)
                  n92 = call "总磷氨氮操作日志.vi"("data in"=w149) -> ()  [unwired: 11 in]
                }
              }
            }
            n93 = local write "数组"(w116) -> ()
          }
        }
      }
    }
    n94 = feedback #5() -> (w100:T8)  [unwired: 1 in]
    n95 = feedback-in #5(w84) -> ()
    n96 = Not Equal?(x=w84, y=w100) -> (x != y?=w101:cluster{"启动模式":bool, "启动参数":bool, "量程":bool})
    n97 = Cluster To Array(cluster=w101) -> (array=w102:bool[])
    n98 = Boolean Array To Number(Boolean array=w102) -> (number=w103:u32)
    n99 = Not Equal To 0?(x=w103) -> (x != 0?=w96:bool)
    n100 = First Call?() -> (First Call?: T/F=w97:bool)
    n101 = Or(x=w96, y=w97) -> (x .or. y?=w95:bool)
    n102 = while {
      tunnel: w95 -> [w241]
      tunnel: w84 -> [w240]
      shift-right: [w239] -> w99
      shift-left: _ -> [w235]
      shift-right: [w238] -> w98
      shift-left: _ -> [w236]
      stop <- TRUE stop-if-true
      n103 = case shown="真" w241 {
        tunnel: [w243 w250] -> w238
        tunnel: [w242 w249] -> w239
        tunnel: w240 -> [_ w244]
        tunnel: w236 -> [w243 _]
        tunnel: w235 -> [w242 _]
        frame False {
        }
        frame True {
          n104 = call "斯坦道XML解析.vi"("参数簇"=w244) -> ("步骤时间"=w245:string[], "步骤名"=w247:string[])  [unwired: 9 in]
          n105 = for {
            tunnel: w247 -> [_] mode=indexing
            tunnel: [w251] -> w248 mode=indexing
            i -> [w251]
          }
          n106 = Build Array(w247, w245) -> (w246:string[][])
          n107 = Transpose 2D Array(2D array=w246) -> (transposed array=w249:string[][])
          n108 = Number To Decimal String(number=w248) -> (decimal integer string=w250:string[])  [unwired: 1 in]
        }
      }
    }
    n109 = global read "VAR总磷氨氮全局变量.vi" "状态告警区"() -> (w85:T3)
    "总磷总氮运行状态" <- w85
    n110 = Unbundle By Name(w85) -> ("日志代码"=w72:u16)
    n111 = feedback-in #6(w72) -> ()
    n112 = feedback #6(w72) -> (w105:u16)
    n113 = Not Equal?(x=w72, y=w105) -> (x != y?=w104:bool)
    n114 = case shown="真" w104 {
      tunnel: w72 -> [_ w254]
      tunnel: w99 -> [_ w261]
      tunnel: w98 -> [_ w260]
      frame False {
      }
      frame True {
        n115 = Subtract(x=w254, y=1) -> (x-y=w252:i32)
        "多列列表框" <- w252
        n116 = Subtract(x=w252, y=5) -> (x-y=w256:i32)
        n117 = property on="多列列表框" class="MCListbox (严格)"("ItemNames"=w261, "RowHdrs[]"=w260) -> (error out=w262:errorcluster)  [unwired: 2 in, 1 out]
        n118 = Greater Or Equal To 0?(x=w256) -> (x >= 0?=w255:bool)
        n119 = property on="多列列表框" class="MCListbox (严格)"(error in=w262) -> (error out=w263:errorcluster, "TopLeft"=w264:T12)  [unwired: 1 in, 1 out]
        n120 = Select(t=w256, s=w255, f=0) -> (s? t:f=w257:i32)
        n121 = Bundle By Name(cluster=w264, "Row"=w257) -> (w265:T12)
        n122 = property on="多列列表框" class="MCListbox (严格)"(error in=w263, "TopLeft"=w265) -> ()  [unwired: 1 in, 2 out]
      }
    }
  }
  n123 = node-c288() -> (w5:T13)  [unwired: 4 in]
  n124 = property class="VI"(reference=w23) -> ("Name"=w16:string)  [unwired: 1 in, 2 out]
  n125 = control-ref of="测量模式下拉列表"() -> (w12:refnum<vi>)
  n126 = control-ref of="量程切换阈值"() -> (w10:refnum<vi>)
  n127 = control-ref of="参数下拉列表"() -> (w13:refnum<vi>)
  n128 = control-ref of="量程下拉列表"() -> (w14:refnum<vi>)
  n129 = control-ref of="备用系数"() -> (w9:refnum<vi>)
  n130 = Open VI Reference(type specifier VI Refnum (for type only)=refnum<vi> refnum, vi path=w30, options=128 ("选项")) -> (vi reference=w28:refnum<vi>, error out=w26:errorcluster)  [unwired: 3 in]
  n131 = control-ref of="公式"() -> (w11:refnum<vi>)
  n132 = timed-loop {
    timing: w5 -> [_]
    timing-out: [_] -> w4
    tunnel: w1 -> [w268]
    stop <- FALSE stop-if-true
    w269 = u16 3 items=["总磷"=1, "氨氮"=3] ("站号")
    # "定时更新"
    n133 = node-c288() -> ()  [unwired: 1 in, 1 out]
    n134 = call "总磷氨氮版本号读取.vi"() -> ("固件版本号"=→"固件版本号":string)  [unwired: 11 in]
    n135 = Bundle By Name(cluster=cluster{"命令":string, "data":variant} {"命令"="", "data"=variant} ("元素"), "命令"="读序列号", "data"=w269) -> (w267:cluster{"命令":string, "data":variant})
    n136 = Enqueue Element(queue=w268, element=w267) -> ()  [unwired: 2 in, 3 out]
    n137 = node-c288() -> ()  [unwired: 1 in, 1 out]
  }
  n138 = call-by-ref "?"(reference=w28, error in=w26) -> (reference out=w24:refnum<vi>, error out=w25:errorcluster)  [unwired: 12 in]
  n139 = Open VI Reference(type specifier VI Refnum (for type only)=refnum<vi> refnum, vi path=w16, options=128 ("选项")) -> (vi reference=w18:refnum<vi>, error out=w20:errorcluster)  [unwired: 3 in]
  n140 = call-by-ref "?"(reference=w18, error in=w20) -> (reference out=w22:refnum<vi>, error out=w21:errorcluster)  [unwired: 12 in]
  n141 = Close Reference(reference=w24, error in (no error)=w25) -> ()  [unwired: 1 out]
  n142 = while {
    tunnel: w34 -> [w277]
    shift-right: [w278] -> _
    shift-left: T4."待机" -> [w279]
    shift-right: [w275] -> _
    shift-left: u32 0 ("等待时间（毫秒）") -> [w276]
    stop <- FALSE stop-if-true
    n143 = Wait (ms)(milliseconds to wait=u32 1000 ("等待时间（毫秒）")) -> ()  [unwired: 1 out]
    n144 = local read "定时启动"() -> (w280:bool)
    n145 = case shown="真" w280 {
      tunnel: w279 -> [_ w288]
      tunnel: [T4."待机" w287] -> w278
      tunnel: w277 -> [_ w286]
      tunnel: w276 -> [_ w285]
      tunnel: [_ w284] -> w275
      frame False {
      }
      frame True {
        n146 = case shown="\"氨氮测量中\"" w288 {
          tunnel: [T4."启动氨氮" w293 w300 w311 w319 w331] -> w287
          tunnel: w286 -> [_ w298 _ w317 _ _]
          tunnel: w285 -> [_ _ _ _ _ w334]
          tunnel: [_ _ _ _ _ w330] -> w284
          frame "待机", Default {
          }
          frame "启动氨氮" {
            n147 = call "总磷氨氮启动命令.vi"("参数"=T16 {"站号"=3, "量程切换"=enum."AUTO", "控制命令"=enum."启动测量", "模式设置"=enum."待机", "测量间隔"=0}) -> ("启动命令"=w291:cluster{"命令":string, "data":variant})  [unwired: 10 in]
            n148 = Enqueue Element(queue=w298, element=w291) -> ()  [unwired: 2 in, 3 out]
            n149 = global read "VAR总磷氨氮全局变量.vi" "状态告警区"() -> (w297:T3)
            n150 = Unbundle By Name(w297) -> ("工作状态"=w296:T7)
            n151 = Not Equal To 0?(x=w296) -> (x != 0?=w295:bool)
            n152 = Select(t=T4."氨氮测量中", s=w295, f=T4."启动氨氮") -> (s? t:f=w293:T4)
          }
          frame "氨氮测量中" {
            n153 = flat-sequence {
              tunnel: [w304] -> w299
              tunnel: [w308] -> w300
              tunnel: w299 -> [w308]
              frame #0 {
                n154 = global read "VAR总磷氨氮全局变量.vi" "状态告警区"() -> (w305:T3)
                n155 = Unbundle By Name(w305) -> ("工作状态"=w306:T7)
                n156 = Equal To 0?(x=w306) -> (x = 0?=w301:bool)
                n157 = Select(t=T4."延时", s=w301, f=T4."氨氮测量中") -> (s? t:f=w304:T4)
              }
              frame #1 {
                n158 = Wait (ms)(milliseconds to wait=u32 5000 ("等待时间（毫秒）")) -> ()  [unwired: 1 out]
              }
            }
          }
          frame "启动总磷" {
            n159 = call "总磷氨氮启动命令.vi"("参数"=T16 {"站号"=1, "量程切换"=enum."AUTO", "控制命令"=enum."启动测量", "模式设置"=enum."待机", "测量间隔"=0}) -> ("启动命令"=w310:cluster{"命令":string, "data":variant})  [unwired: 10 in]
            n160 = Enqueue Element(queue=w317, element=w310) -> ()  [unwired: 2 in, 3 out]
            n161 = global read "VAR总磷氨氮全局变量.vi" "状态告警区"() -> (w312:T3)
            n162 = Unbundle By Name(w312) -> ("工作状态"=w313:T7)
            n163 = Not Equal To 0?(x=w313) -> (x != 0?=w314:bool)
            n164 = Select(t=T4."总磷测量中", s=w314, f=T4."启动总磷") -> (s? t:f=w311:T4)
          }
          frame "总磷测量中" {
            n165 = flat-sequence {
              tunnel: [w321] -> w318
              tunnel: [w327] -> w319
              tunnel: w318 -> [w327]
              frame #0 {
                n166 = global read "VAR总磷氨氮全局变量.vi" "状态告警区"() -> (w324:T3)
                n167 = Unbundle By Name(w324) -> ("工作状态"=w325:T7)
                n168 = Equal To 0?(x=w325) -> (x = 0?=w320:bool)
                n169 = Select(t=T4."延时", s=w320, f=T4."总磷测量中") -> (s? t:f=w321:T4)
              }
              frame #1 {
                n170 = Wait (ms)(milliseconds to wait=u32 5000 ("等待时间（毫秒）")) -> ()  [unwired: 1 out]
              }
            }
          }
          frame "延时" {
            n171 = local read "设置值"() -> (w333:dbl)
            n172 = Increment(x=w334) -> (x+1=w330:u32)
            n173 = Greater Or Equal?(x=w330, y=w333) -> (x >= y?=w332:bool)
            n174 = Select(t=T4."待机", s=w332, f=T4."延时") -> (s? t:f=w331:T4)
          }
        }
      }
    }
  }
  n175 = while {
    tunnel: w34 -> [w341]
    tunnel: w14 -> [w340]
    tunnel: w13 -> [w339]
    tunnel: w12 -> [w338]
    tunnel: w11 -> [w337]
    tunnel: w10 -> [w336]
    tunnel: w9 -> [w335]
    tunnel: w7 -> [_]
    stop <- FALSE stop-if-true
    n176 = event shown="[9] \"标液浓度1\", \"标液浓度2\", \"标液浓度3\", \"标液浓度4\", \"标液浓度5\", \"样品1 F0\", \"样品1 F1\", \"样品2 F1\", \"样品2 F0\", \"样品3 F1\", \"样品3 F0\", \"样品4 F0\", \"样品4 F1\", \"样品5 F0\", \"样品5 F1\", \"精度\", \"公式.X^2\", \"公式.X\", \"公式.b\", \"量程切换阈值.阈值\", \"量程切换阈值.标液浓度\", \"备用系数.量程上限\", \"备用系数.量程下限\", \"备用系数.检出限\", \"备用系数.精度\", \"测量吸光度1\", \"测量吸光度2\", \"测量吸光度3\", \"测量吸光度4\", \"测量吸光度5\": 鼠标按下" {
      selector: _ -> [_ _ _ _ _ _ _ _ _ _ _ _ _ _ _ _]
      dyn-events: _ -> [_ _ _ _ _ _ _ _ _ _ _ _ _ _ _ _]
      timeout: _ -> [_ _ _ _ _ _ _ _ _ _ _ _ _ _ _ _]
      tunnel: w341 -> [_ w345 _ w356 w358 _ _ _ _ _ _ _ _ _ _ _]
      tunnel: w340 -> [_ _ _ _ _ _ _ _ _ _ w416 _ w436 w445 _ _]
      tunnel: w339 -> [_ _ _ _ _ _ _ _ _ _ w414 _ w434 w447 w455 w462]
      tunnel: w338 -> [_ _ _ _ _ _ _ _ _ _ w415 _ w435 w446 _ _]
      tunnel: w337 -> [_ _ _ _ _ _ _ _ _ _ w410 _ _ _ _ _]
      tunnel: w336 -> [_ _ _ _ _ _ _ _ _ _ _ _ w430 _ _ _]
      tunnel: w335 -> [_ _ _ _ _ _ _ _ _ _ _ _ _ _ w453 _]
      event Timeout {
        n177 = event-data() -> ()  [unwired: 1 in, 3 out]
      }
      event "手动启动": Value Change {
        n178 = event-data() -> ()  [unwired: 1 in, 6 out]
        n179 = call "总磷氨氮启动参数对话框.vi"() -> ("确认"=w343:bool, "元素"=w344:cluster{"命令":string, "data":variant})  [unwired: 10 in]
        n180 = case shown="真" w343 {
          tunnel: w345 -> [_ w347]
          tunnel: w344 -> [_ w346]
          frame False {
          }
          frame True {
            n181 = Enqueue Element(queue=w347, element=w346) -> ()  [unwired: 2 in, 3 out]
          }
        }
      }
      event "定时启动": Mouse Down {
        n182 = event-data() -> ()  [unwired: 1 in, 6 out]
        n183 = call "定时启动对话框.vi"() -> ("设置值"=→"设置值":dbl, "确定输出"=→"定时启动":bool)  [unwired: 10 in]
      }
      event "单步测试": Value Change {
        w351 = u16 1 items=["总磷"=1, "氨氮"=3] ("站号")
        n184 = event-data() -> ()  [unwired: 1 in, 6 out]
        n185 = Bundle("站号"=w351, "总磷氨氮调试"="总磷氨氮调试") -> (w350:cluster{"站号":u16, "总磷氨氮调试":u16[]})  [unwired: 1 in]
        n186 = Bundle By Name(cluster=cluster{"命令":string, "data":variant} {"命令"="", "data"=variant} ("元素"), "命令"="debug", "data"=w350) -> (w353:cluster{"命令":string, "data":variant})
        n187 = Enqueue Element(queue=w356, element=w353) -> ()  [unwired: 2 in, 3 out]
      }
      event "停止": Value Change {
        n188 = event-data() -> ()  [unwired: 1 in, 6 out]
        n189 = Enqueue Element(queue=w358, element=cluster{"命令":string, "data":variant} {"命令"="启动", "data"=variant(cluster{"站号":u16, "控制命令输出":u16[]} {"站号"=1, "控制命令输出"=[2816]})} ("元素")) -> ()  [unwired: 2 in, 3 out]
      }
      event "设置": Value Change {
        n190 = event-data() -> ()  [unwired: 1 in, 6 out]
        n191 = property on="窗格" class="Pane"("Origin"=T5 {"Horizontal"=0, "Vertical"=528} ("原点")) -> ()  [unwired: 2 in, 2 out]
      }
      event "返回": Value Change {
        n192 = event-data() -> ()  [unwired: 1 in, 6 out]
        n193 = property on="窗格" class="Pane"("Origin"=T5 {"Horizontal"=0, "Vertical"=0} ("原点")) -> ()  [unwired: 2 in, 2 out]
      }
      event "标液浓度1", "测量吸光度1", "测量吸光度2", "标液浓度2", "测量吸光度3", "标液浓度3", "测量吸光度4", "标液浓度4", "测量吸光度5", "标液浓度5", "样品1启用", "样品3启用", "样品4启用", "样品5启用", "样品2启用", "模型", "method", "精度": Value Change {
        n194 = event-data() -> ()  [unwired: 1 in, 6 out]
        n195 = Replace Array Subset(array=dbl[] [0.0, 0.0, 0.0, 0.0, 0.0] ("数组"), new element #1="标液浓度1", new element #2="标液浓度2", new element #3="标液浓度3", new element #4="标液浓度4", new element #5="标液浓度5") -> (w367:dbl[])  [unwired: 5 in]
        n196 = Replace Array Subset(array=dbl[] [0.0, 0.0, 0.0, 0.0, 0.0] ("数组"), new element #1="测量吸光度1", new element #2="测量吸光度2", new element #3="测量吸光度3", new element #4="测量吸光度4", new element #5="测量吸光度5") -> (w366:dbl[])  [unwired: 5 in]
        n197 = Replace Array Subset(array=bool[] [FALSE, FALSE, FALSE, FALSE, FALSE] ("数组"), new element #1="样品1启用", new element #2="样品2启用", new element #3="样品3启用", new element #4="样品4启用", new element #5="样品5启用") -> (w365:bool[])  [unwired: 5 in]
        n198 = call "线性公式.vi"("精度"="精度", "模型"="模型", "method"="method", "启用"=w365, "监测浓度"=w366, "标液浓度"=w367) -> ("XY图"=→"XY图":cluster{"X Values":dbl[], "Y Values":dbl[]}[], "r^2"=→"r^2":dbl, "拟合方程"=→"拟合公式":string)  [unwired: 3 in]
      }
      event "样品1 F0", "样品1 F1", "样品2 F1", "样品2 F0", "样品3 F1", "样品3 F0", "样品4 F0", "样品4 F1", "样品5 F1", "样品5 F0": Value Change {
        n199 = event-data() -> ()  [unwired: 1 in, 6 out]
        n200 = formula code="E=log(F0/F1);"("F0"="样品5 F0", "F1"="样品5 F1") -> ("E"=w391:dbl)
        n201 = formula code="E=log(F0/F1);"("F0"="样品4 F0", "F1"="样品4 F1") -> ("E"=w390:dbl)
        n202 = formula code="E=log(F0/F1);"("F0"="样品3 F0", "F1"="样品3 F1") -> ("E"=w389:dbl)
        n203 = formula code="E=log(F0/F1);"("F0"="样品2 F0", "F1"="样品2 F1") -> ("E"=w388:dbl)
        n204 = formula code="E=log(F0/F1);"("F0"="样品1 F0", "F1"="样品1 F1") -> ("E"=w392:dbl)
        n205 = property on="测量吸光度5" class="DigNum (严格)"("Val(Sgnl)"=w391) -> ()  [unwired: 2 in, 2 out]
        n206 = property on="测量吸光度4" class="DigNum (严格)"("Val(Sgnl)"=w390) -> ()  [unwired: 2 in, 2 out]
        n207 = property on="测量吸光度3" class="DigNum (严格)"("Val(Sgnl)"=w389) -> ()  [unwired: 2 in, 2 out]
        n208 = property on="测量吸光度2" class="DigNum (严格)"("Val(Sgnl)"=w388) -> ()  [unwired: 2 in, 2 out]
        n209 = property on="测量吸光度1" class="DigNum (严格)"("Val(Sgnl)"=w392) -> ()  [unwired: 2 in, 2 out]
      }
      event "标液浓度1", "标液浓度2", "标液浓度3", "标液浓度4", "标液浓度5", "样品1 F0", "样品1 F1", "样品2 F1", "样品2 F0", "样品3 F1", "样品3 F0", "样品4 F0", "样品4 F1", "样品5 F0", "样品5 F1", "精度", "公式.X^2", "公式.X", "公式.b", "量程切换阈值.阈值", "量程切换阈值.标液浓度", "备用系数.量程上限", "备用系数.量程下限", "备用系数.检出限", "备用系数.精度", "测量吸光度1", "测量吸光度2", "测量吸光度3", "测量吸光度4", "测量吸光度5": Mouse Down {
        n210 = event-data() -> ("CtlRef"=w406:refnum<vi>)  [unwired: 1 in, 5 out]
        n211 = property class="DigNum (严格)"(reference=w406) -> (reference out=w404:refnum<vi>, "Value"=w405:dbl)  [unwired: 1 in, 1 out]
        n212 = call "数字键盘.vi"("OldNumber"=w405) -> ("NewNumber"=w403:sgl)
        n213 = property class="DigNum (严格)"(reference=w404, "Val(Sgnl)"=w403) -> ()  [unwired: 1 in, 2 out]
      }
      event "读公式": Value Change {
        n214 = event-data() -> ()  [unwired: 1 in, 6 out]
        n215 = property class="Enum (严格)"(reference=w414) -> ("Value"=w413:enum16{"氨氮", "总磷"})  [unwired: 1 in, 2 out]
        n216 = property class="Enum (严格)"(reference=w415) -> ("Value"=w412:enum16{"水样测量", "空白核查", "标样核查", "盲样测试", "加标回收"})  [unwired: 1 in, 2 out]
        n217 = property class="Enum (严格)"(reference=w416) -> ("Value"=w411:enum16{"低量程", "高量程"})  [unwired: 1 in, 2 out]
        n218 = call "总磷氨氮公式读取.vi"("量程"=w411, "测量模式"=w412, "测量参数"=w413) -> ("error out"=w408:errorcluster, "公式"=w409:cluster{"X^2":dbl, "X":dbl, "b":dbl})  [unwired: 7 in]
        n219 = property class="Clust (严格)"(reference=w410, "Value"=w409) -> ()  [unwired: 1 in, 2 out]
        n220 = case shown="错误" w408 {
          tunnel: ["读取成功" ("消息") "读取失败" ("消息")] -> w407
          frame No Error {
          }
          frame Error {
          }
        }
        n221 = One Button Dialog(message=w407) -> ()  [unwired: 1 in, 1 out]
      }
      event "写公式": Value Change {
        n222 = event-data() -> ()  [unwired: 1 in, 6 out]
        n223 = call "总磷氨氮公式写入.vi"("公式"="公式", "量程"="量程下拉列表", "测量模式"="测量模式下拉列表", "测量参数"="参数下拉列表") -> ("error out"=w419:errorcluster)  [unwired: 7 in]
        n224 = case shown="无错误" w419 {
          tunnel: ["写入成功" ("消息") "写入失败" ("消息")] -> w420
          frame No Error {
          }
          frame Error {
          }
        }
        n225 = One Button Dialog(message=w420) -> ()  [unwired: 1 in, 1 out]
      }
      event "量程切换阈值读取": Value Change {
        n226 = event-data() -> ()  [unwired: 1 in, 6 out]
        n227 = property class="Enum (严格)"(reference=w434) -> ("Value"=w433:enum16{"氨氮", "总磷"})  [unwired: 1 in, 2 out]
        n228 = property class="Enum (严格)"(reference=w435) -> ("Value"=w432:enum16{"水样测量", "空白核查", "标样核查", "盲样测试", "加标回收"})  [unwired: 1 in, 2 out]
        n229 = property class="Enum (严格)"(reference=w436) -> ("Value"=w431:enum16{"低量程", "高量程"})  [unwired: 1 in, 2 out]
        n230 = call "总磷氨氮量程读取.vi"("量程"=w431, "测量模式"=w432, "测量参数"=w433) -> ("error out"=w427:errorcluster, "量程切换阈值"=w429:cluster{"阈值":dbl, "标液浓度":dbl})  [unwired: 7 in]
        n231 = property class="Clust (严格)"(reference=w430, "Value"=w429) -> ()  [unwired: 1 in, 2 out]
        n232 = case shown="错误" w427 {
          tunnel: ["读取成功" ("消息") "读取失败" ("消息")] -> w428
          frame No Error {
          }
          frame Error {
          }
        }
        n233 = One Button Dialog(message=w428) -> ()  [unwired: 1 in, 1 out]
      }
      event "量程切换阈值写入": Value Change {
        n234 = event-data() -> ()  [unwired: 1 in, 6 out]
        n235 = property class="Enum (严格)"(reference=w447) -> ("Value"=w444:enum16{"氨氮", "总磷"})  [unwired: 1 in, 2 out]
        n236 = property class="Enum (严格)"(reference=w446) -> ("Value"=w443:enum16{"水样测量", "空白核查", "标样核查", "盲样测试", "加标回收"})  [unwired: 1 in, 2 out]
        n237 = property class="Enum (严格)"(reference=w445) -> ("Value"=w442:enum16{"低量程", "高量程"})  [unwired: 1 in, 2 out]
        n238 = call "总磷氨氮量程写入.vi"("量程切换阈值"="量程切换阈值", "量程"=w442, "测量模式"=w443, "测量参数"=w444) -> ("error out"=w439:errorcluster)  [unwired: 7 in]
        n239 = case shown="无错误" w439 {
          tunnel: ["写入成功" ("消息") "写入失败" ("消息")] -> w440
          frame No Error {
          }
          frame Error {
          }
        }
        n240 = One Button Dialog(message=w440) -> ()  [unwired: 1 in, 1 out]
      }
      event "备用系数读取": Value Change {
        n241 = event-data() -> ()  [unwired: 1 in, 6 out]
        n242 = property class="Enum (严格)"(reference=w455) -> ("Value"=w454:enum16{"氨氮", "总磷"})  [unwired: 1 in, 2 out]
        n243 = call "总磷氨氮备用系数读取.vi"("测量参数"=w454) -> ("error out"=w450:errorcluster, "备用系数"=w452:T1)  [unwired: 9 in]
        n244 = property class="Clust (严格)"(reference=w453, "Value"=w452) -> ()  [unwired: 1 in, 2 out]
        n245 = case shown="错误" w450 {
          tunnel: ["读取成功" ("消息") "读取失败" ("消息")] -> w451
          frame No Error {
          }
          frame Error {
          }
        }
        n246 = One Button Dialog(message=w451) -> ()  [unwired: 1 in, 1 out]
      }
      event "备用系数写入": Value Change {
        n247 = event-data() -> ()  [unwired: 1 in, 6 out]
        n248 = property class="Enum (严格)"(reference=w462) -> ("Value"=w461:enum16{"氨氮", "总磷"})  [unwired: 1 in, 2 out]
        n249 = call "总磷氨氮备用系数写入.vi"("备用系数"="备用系数", "测量参数"=w461) -> ("error out"=w458:errorcluster)  [unwired: 9 in]
        n250 = case shown="无错误" w458 {
          tunnel: ["写入成功" ("消息") "写入失败" ("消息")] -> w459
          frame No Error {
          }
          frame Error {
          }
        }
        n251 = One Button Dialog(message=w459) -> ()  [unwired: 1 in, 1 out]
      }
    }
  }
  n252 = while {
    tunnel: w34 -> [w480]
    tunnel: w35 -> [_]
    shift-right: [w474] -> _
    shift-left: enum16{"氨氮", "总磷"}."氨氮" ("枚举") -> [w475]
    stop <- FALSE stop-if-true
    w473 = u16 3 items=["总磷"=1, "氨氮"=3] ("站号")
    # "试剂填充 172 \n管路清洗108\n氨氮92\n总磷131\n总磷海水147\n总氮76\n总氮海水92"
    n253 = Wait (ms)(milliseconds to wait=u32 1000 ("等待时间（毫秒）")) -> ()  [unwired: 1 out]
    n254 = Bundle By Name(cluster=cluster{"命令":string, "data":variant} {"命令"="", "data"=variant} ("元素"), "命令"="读状态告警区", "data"=w473) -> (w482:cluster{"命令":string, "data":variant})
    n255 = global read "VAR总磷氨氮全局变量.vi" "状态告警区"() -> (w471:T3)
    n256 = Bundle By Name(cluster=cluster{"命令":string, "data":variant} {"命令"="", "data"=variant} ("元素"), "命令"="读测量数据区", "data"=w473) -> (w478:cluster{"命令":string, "data":variant})
    n257 = Unbundle By Name(w471) -> ("系统时间"=w470:timestamp)
    n258 = Enqueue Element(queue=w480, element=w482) -> (queue out=w476:refnum<queue>)  [unwired: 2 in, 2 out]
    n259 = Enqueue Element(queue=w476, element=w478) -> (queue out=w472:refnum<queue>)  [unwired: 2 in, 2 out]
    n260 = Get Date/Time In Seconds() -> (seconds since 1Jan1904=w469:timestamp)
    n261 = Subtract(x=w469, y=w470) -> (x-y=w468:dbl)
    n262 = Absolute Value(x=w468) -> (abs(x)=w467:dbl)
    n263 = Greater Or Equal?(x=w467, y=120.0) -> (x >= y?=w465:bool)
    n264 = case shown="真" w465 {
      tunnel: w472 -> [_ w487]
      frame False {
      }
      frame True {
        n265 = call "总磷氨氮启动命令.vi"("参数"=T17 {"站号"=3, "量程切换"=enum."AUTO", "控制命令"=enum."校时", "模式设置"=enum."待机", "测量间隔"=0}) -> ("启动命令"=w486:cluster{"命令":string, "data":variant})  [unwired: 10 in]
        n266 = Enqueue Element(queue=w487, element=w486) -> ()  [unwired: 2 in, 3 out]
      }
    }
    n267 = Increment(x=w475) -> (x+1=w474:enum16{"氨氮", "总磷"})
  }
  n268 = Close Reference(reference=w22, error in (no error)=w21) -> ()  [unwired: 1 out]
  n269 = node-c288(w4) -> ()  [unwired: 1 out]
